vi "Get Selected XNET Channels.vi"(6 "Add Info?":bool, 8 "error in (no error)":errorcluster, 9 "Node Ptr":u64 format="%.0x", 10 "XNET Cluster":refnum<k21>, 11 "Tree In":refnum<vi>) -> (0 "error out":errorcluster, 2 "XNET Signal Names":refnum<k21>[](array[refnum]), 3 "Tree Out":refnum<vi>)   [LabVIEW 2019, in "Protection and Counter Addon System Explorer.lvlib"]
uses:
  Protection and Counter Addon System Explorer.lvlib
  <resource>/objmgr/xnet.rc
  <vilib>/NI VeriStand/Custom Device API/Custom Device API.lvlib
panel:
  # "OUTPUTS"
  # "INPUTS"
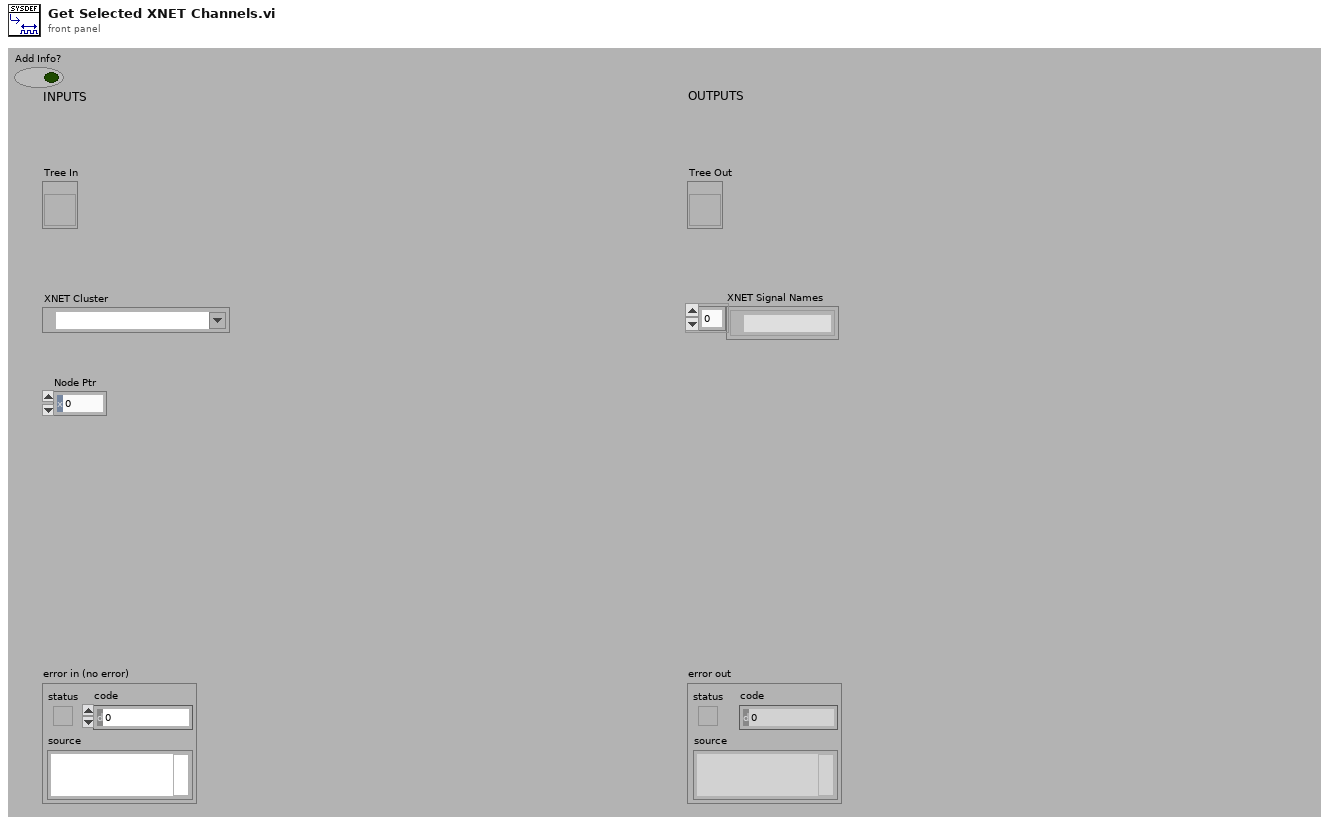
[diagram p1: front panel]
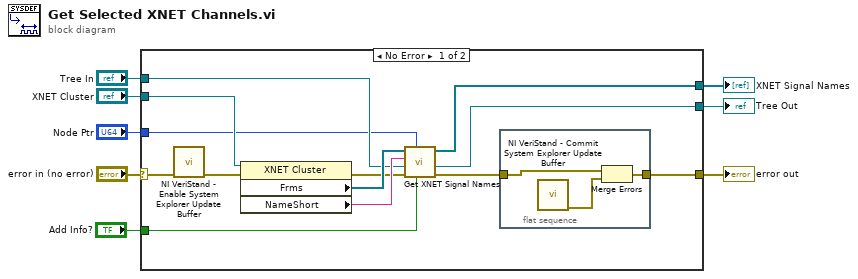
[diagram p0: block diagram]
diagram:
  n1 = case shown="No Error" "error in (no error)" {
    selector: "error in (no error)" -> [w14 w26]
    tunnel: [w12 w26] -> w7
    tunnel: "XNET Cluster" -> [w21 _]
    tunnel: [w16 _] -> w5
    tunnel: "Tree In" -> [w15 w25]
    tunnel: [w18 w25] -> w3
    tunnel: "Node Ptr" -> [w10 _]
    tunnel: "Add Info?" -> [w11 _]
    frame No Error {
      n2 = call <vilib>:"NI VeriStand - Enable System Explorer Update Buffer.vi"("error in (no error)"=w14) -> ("error out"=w9:errorcluster)  [unwired: 10 in]
      n3 = property class="XNET Cluster"(reference=w21, error in=w9) -> (error out=w17:errorcluster, "Frms"=w20:refnum<k21>[], "NameShort"=w19:string)  [unwired: 1 out]
      n4 = call "Get XNET Signal Names.vi"("Add Info?"=w11, "Parent Ref in"=w10, "error in"=w17, "Tree In"=w15, "Parent"=w19, "Frms"=w20) -> ("error out"=w13:errorcluster, "Tree Out"=w18:refnum<vi>, "XNET Signal Names"=w16:refnum<k21>[])  [unwired: 3 in]
      n5 = flat-sequence {
        tunnel: w13 -> [w23]
        tunnel: [w22] -> w12
        frame #0 {
          n6 = call <vilib>:"NI VeriStand - Commit System Explorer Update Buffer.vi"() -> ("error out"=w24:errorcluster)  [unwired: 11 in]
          n7 = Merge Errors(w23, w24) -> (w22:errorcluster)
        }
      }
    }
    frame Error {
    }
  }
  "error out" <- w7
  "XNET Signal Names" <- w5
  "Tree Out" <- w3
